vi "Set Slave ID.vi"(8 "error in (no error)":errorcluster, 10 "Slave ID":u8=1, 11 "MB_TCP_Master in":refnum<class "MB_Master_TCP.lvclass">) -> (0 "error out":errorcluster, 3 "MB_TCP_Master out":refnum<class "MB_Master_TCP.lvclass">)   [LabVIEW 2016, in "MB Master.lvlib" / "MB_Master_TCP.lvclass"]
uses:
  MB_Master_TCP.lvclass
  MB_Master_TCP.lvclass/MB_Master_TCP.ctl
  MB_ADU/MB_ADU.lvclass/MB_ADU.ctl
  MB_ADU_TCP/MB_ADU_TCP.lvclass
  C:/Users/illogicdev/Desktop/IGUS/20190906-1xdryveD1+LABview+ModbusTCP(Gateway)/IgusPositioningSystem Folder/Modules/Libraries/Modbus-Master/MB_ADU/MB_ADU.lvclass
  MB_ADU/MB_ADU.lvclass
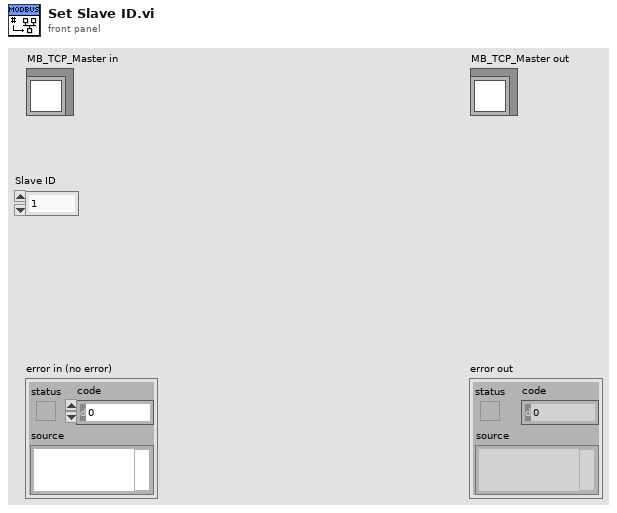
[diagram p1: front panel]
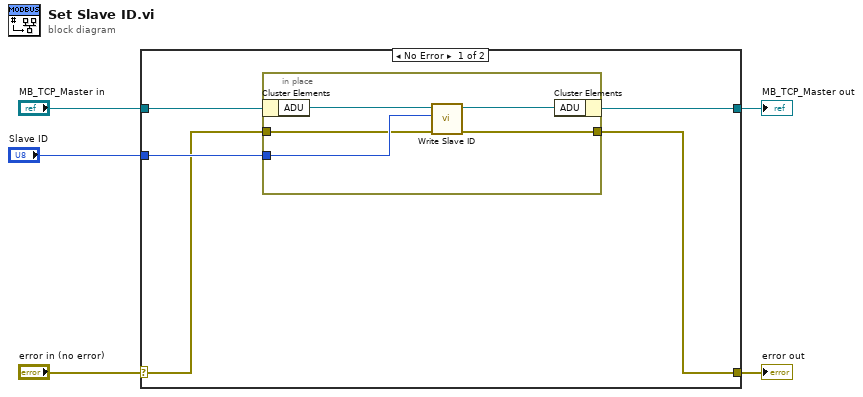
[diagram p0: block diagram]
diagram:
  n1 = case shown="No Error" "error in (no error)" {
    selector: "error in (no error)" -> [w7 w17]
    tunnel: [w6 w17] -> w4
    tunnel: [w8 w16] -> w2
    tunnel: "MB_TCP_Master in" -> [w10 w16]
    tunnel: "Slave ID" -> [w9 _]
    frame No Error {
      n2 = in-place {
        in-place-border: w9 -> [w13]
        in-place-border: w7 -> [w12]
        in-place-border: [w11] -> w6
        n3 = in-place-cluster #1(w10) -> ("ADU"=w15:refnum<class "MB_ADU_TCP.lvclass">)
        n4 = call "Write Slave ID.vi"("error in (no error)"=w12, "Slave Address"=w13, "MB_ADU_Serial in"=w15) -> ("error out"=w11:errorcluster, "MB_ADU_Serial out"=w14:refnum<class "MB_ADU_TCP.lvclass">)  [unwired: 7 in]
        n5 = in-place-cluster #1("ADU"=w14) -> (w8:refnum<class "MB_Master_TCP.lvclass">)
      }
    }
    frame Error {
    }
  }
  "error out" <- w4
  "MB_TCP_Master out" <- w2
